vi "GenerateEventBuildingItem.vi"(9 "ProjectItem":refnum<class "ProjectItem.lvclass">, 11 "BuildingItem":refnum<user-event>) -> ()   [LabVIEW 2019, in "SolutionBuilder.lvlib" / "ProjectItem.lvclass"]
uses:
  ProjectItem.lvclass
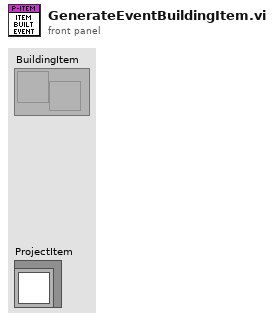
[diagram p1: front panel]
types:
  T1 = cluster{"Build spec name":string, "Target":string, "Owning lib name":string, "Result":string}
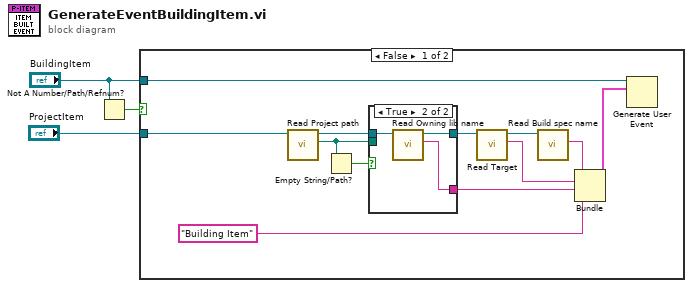
[diagram p0: block diagram]
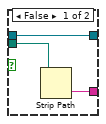
[diagram p2: hidden frame]
diagram:
  n1 = Not A Number/Path/Refnum?(number/path/refnum="BuildingItem") -> (NaN/Path/Refnum?=w1:bool)
  n2 = case shown="False" w1 {
    tunnel: "ProjectItem" -> [w4 _]
    tunnel: "BuildingItem" -> [w13 _]
    frame False {
      n3 = call "Read Project path.vi"("ProjectItem in"=w4) -> ("Project path"=w7:path, "ProjectItem out"=w8:refnum<class "ProjectItem.lvclass">)  [unwired: 9 in]
      n4 = Empty String/Path?(string/path=w7) -> (empty?=w6:bool)
      n5 = case shown="True" w6 {
        tunnel: w8 -> [w17 w21]
        tunnel: [w18 w19] -> w9
        tunnel: [w17 w20] -> w10
        tunnel: w7 -> [w16 _]
        frame False {
          n6 = Strip Path(path=w16) -> (name=w18:string)  [unwired: 1 out]
        }
        frame True {
          n7 = call "Read Owning lib name.vi"("ProjectItem in"=w21) -> ("Owning lib name"=w19:string, "ProjectItem out"=w20:refnum<class "ProjectItem.lvclass">)  [unwired: 9 in]
        }
      }
      n8 = call "Read Target.vi"("ProjectItem in"=w10) -> ("Target"=w11:string, "ProjectItem out"=w12:refnum<class "ProjectItem.lvclass">)  [unwired: 9 in]
      n9 = call "Read Build spec name.vi"("ProjectItem in"=w12) -> ("Build spec name"=w15:string)  [unwired: 9 in, 1 out]
      n10 = Bundle("Build spec name"=w15, "Target"=w11, "Owning lib name"=w9, "Result"="Building Item") -> (w14:T1)  [unwired: 1 in]
      n11 = Generate User Event(user event=w13, event data cluster=w14) -> ()  [unwired: 2 in, 2 out]
    }
    frame True {
    }
  }
